vi "Teleop.vi"(10 "Match Info":T1={"Autonomous Elapsed Seconds"=0.0, "TeleOp Elapsed Seconds"=0.0, "Disabled Elapsed Seconds"=0.0, "Visited Autonomous"=FALSE, "Visited TeleOp"=FALSE, "Visited Disabled"=FALSE, "Autonomous Settings"={"Autonomous Style"=enum."Independent", "VI Refnum"=refnum}}, 11 "Call Context":T2) -> ()   [LabVIEW 2019]
doc: "This VI is called for each TeleOp packet received from the DS where the robot is not disabled. It is often used to read from the joysticks and update I/O or to update setpoints for timed control loops. It should complete and return within 20 milliseconds or it may miss DS packets."
uses:
  <vilib>/Rock Robotics/WPI/DriverStation/WPI_DriverStationDerivedRobotMode.ctl
  <vilib>/Rock Robotics/WPI/DriverStation/WPI_DriverStationMatch Info.ctl
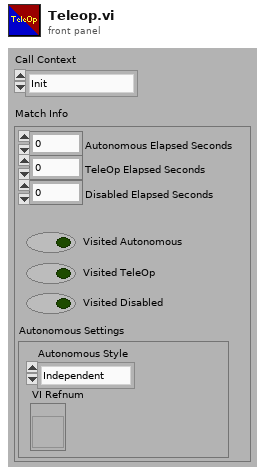
[diagram p1: front panel]
types:
  T1 = typedef "WPI_DriverStationMatch Info.ctl" = cluster{"Autonomous Elapsed Seconds":dbl, "TeleOp Elapsed Seconds":dbl, "Disabled Elapsed Seconds":dbl, "Visited Autonomous":bool, "Visited TeleOp":bool, "Visited Disabled":bool, "Autonomous Settings":cluster{"Autonomous Style":enum16{"Iterative", "Independent"}, "VI Refnum":refnum<vi>}}
  T2 = typedef "WPI_DriverStationDerivedRobotMode.ctl" = enum16{"Init", "Execute", "Stop"}
  T3 = typedef "Joystick_Controls.ctl" = cluster{"Pilot Left Joystick X":dbl, "Pilot Left Joystick Y":dbl, "Pilot A Button":bool, "Pilot B Button":bool, "Pilot X Button":bool, "Pilot Y Button":bool, "Pilot Left Bumper":bool, "Pilot Right Bumper":bool, "Pilot View Button":bool, "Pilot Menu Button":bool, "Pilot Left Joystick Press":bool, "Pilot Right Joystick Press":bool, "Pilot Left Trigger":dbl, "Pilot Right Joystick X":dbl, "Pilot Right Joystick Y":dbl, "Pilot Right Trigger":dbl, "Copilot Left Joystick X":dbl, "Copilot Left Joystick Y":dbl, "Copilot A Button":bool, "Copilot B Button":bool, "Copilot X Button":bool, "Copilot Y Button":bool, "Copilot Left Bumper":bool, "Copilot Right Bumper":bool, "Copilot View Button":bool, "Copilot Menu Button":bool, "Copilot Left Joystick Press":bool, "Copilot Right Joystick Press":bool, "Copilot Left Trigger":dbl, "Copilot Right Joystick X":dbl, "Copilot Right Joystick Y":dbl, "Copilot Right Trigger":dbl, "Pilot D-pad North":bool, "Pilot D-pad South":bool, "Pilot D-pad East":bool, "Pilot D-pad West":bool, "Pilot D-pad NE ":bool, "Pilot D-pad SE":bool, "Pilot D-pad SW":bool, "Pilot D-pad NW":bool, "CoPilot D-pad North":bool, "CoPilot D-pad South":bool, "CoPilot D-pad East":bool, "CoPilot D-pad West":bool, "CoPilot D-pad NE":bool, "CoPilot D-pad SE":bool, "CoPilot D-pad SW":bool, "CoPilot D-pad NW":bool, "Pilot Left Trigger Pressed":bool, "Pilot Right Trigger Pressed":bool, "CoPilot Left Trigger Pressed":bool, "CoPilot Right Trigger Pressed":bool}
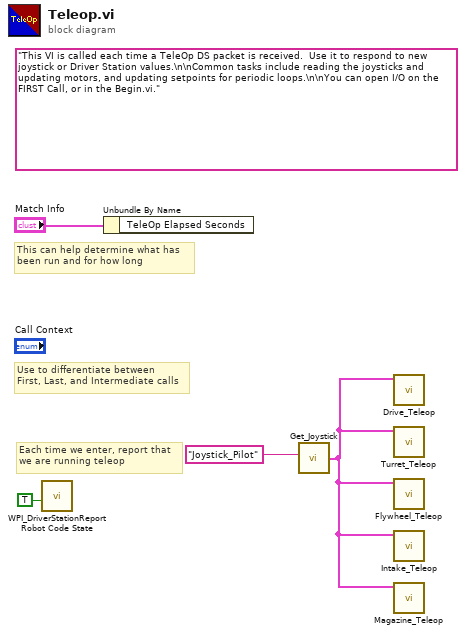
[diagram p0: block diagram]
diagram:
  (unwired) "This VI is called each time a TeleOp DS packet is received.  Use it to respond to new joystick or Driver Station values.\n\nCommon tasks include reading the joysticks and updating motors, and updating setpoints for periodic loops.\n\nYou can open I/O on the FIRST Call, or in the Begin.vi."
  # "Each time we enter, report that\nwe are running teleop"
  # "Use to differentiate between\nFirst, Last, and Intermediate calls"
  # "This can help determine what has\nbeen run and for how long"
  n1 = call <vilib>:"WPI_DriverStationReport Robot Code State.vi"("TeleOp"=TRUE ("Autonomous")) -> ()  [unwired: 10 in, 1 out]
  n2 = Unbundle By Name("Match Info") -> ()  [unwired: 1 out]
  n3 = call "Get_Joystick.vi"("Joystick_One"="Joystick_Pilot") -> ("Joystick_Out"=w1:T3)  [unwired: 6 in]
  n4 = call "Drive_Teleop.vi"("Joystick_Out"=w1) -> ()  [unwired: 4 in]
  n5 = call "Turret_Teleop.vi"("Joystick_IN"=w1) -> ()  [unwired: 11 in]
  n6 = call "Flywheel_Teleop.vi"("Joystick_IN"=w1) -> ()  [unwired: 11 in]
  n7 = call "Intake_Teleop.vi"("Joystick_In"=w1) -> ()  [unwired: 11 in]
  n8 = call "Magazine_Teleop.vi"("Joystick Controls"=w1) -> ()  [unwired: 11 in]
